vi "ConvertRunModesBack.vi"(8 "Error In":errorcluster, 11 "Run Modes in":string[](array[string])) -> (0 "Error Out":errorcluster, 3 "Item Symbols Out":i32[](array[numeric]))   [LabVIEW 2011]
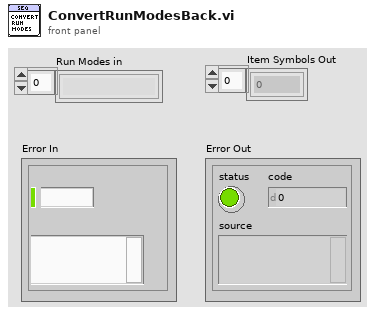
[diagram p1: front panel]
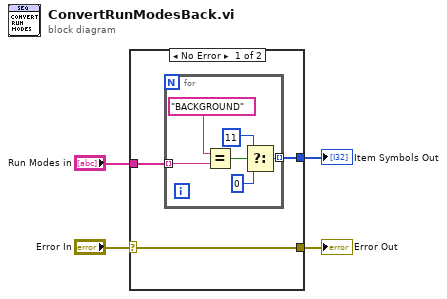
[diagram p0: block diagram]
diagram:
  n1 = case shown="No Error" "Error In" {
    selector: "Error In" -> [w7 w14]
    tunnel: [w7 w14] -> w3
    tunnel: "Run Modes in" -> [w6 _]
    tunnel: [w5 _] -> w1
    frame No Error {
      n2 = for {
        tunnel: w6 -> [w12] mode=indexing
        tunnel: [w8] -> w5 mode=indexing
        n3 = Equal?(x="BACKGROUND" ("Queue Name In"), y=w12) -> (x = y?=w11:bool)
        n4 = Select(t=11 ("y"), s=w11, f=0 ("y")) -> (s? t:f=w8:i32)
      }
    }
    frame Error {
    }
  }
  "Item Symbols Out" <- w1
  "Error Out" <- w3
